vi "CAN wait.vi"(4 "error in (no error)":errorcluster, 5 "Timeout":i32=1000, 6 "Cob ID":u32, 7 "CANopen in":refnum<class "CANopen.lvclass">) -> (0 "error out":errorcluster, 1 "Timeout?":bool, 2 "Data":variant, 3 "CANopen out":refnum<class "CANopen.lvclass">)   [LabVIEW 2017, in "canopen.lvlib" / "CANopen.lvclass"]
doc: "Waits until a specific COB-ID is sent or a specific timeout is elapsed. This VI is <B>blocking</B>!"
uses:
  CANopen.lvclass
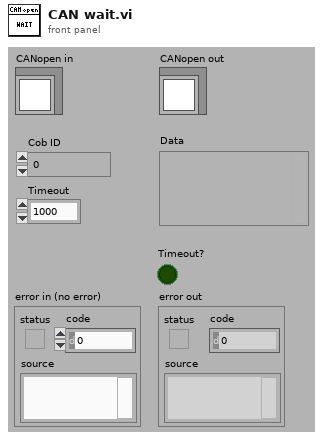
[diagram p1: front panel]
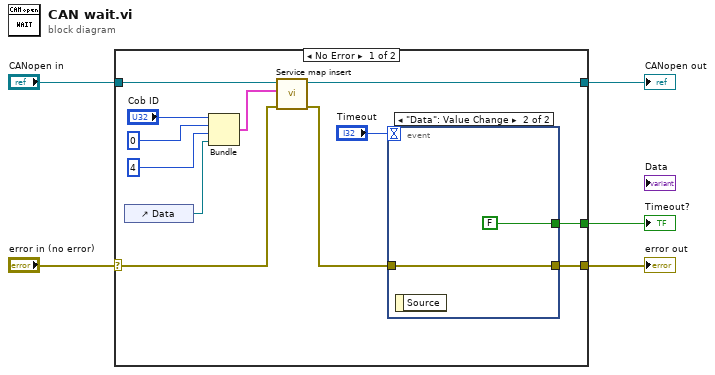
[diagram p0: block diagram]
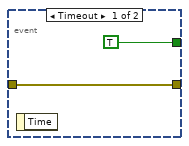
[diagram p2: hidden frame]
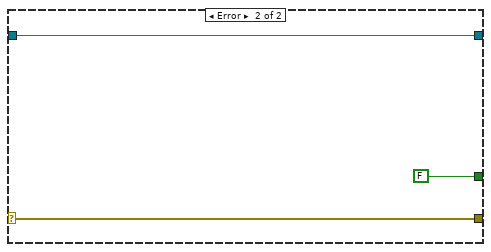
[diagram p3: hidden frame]
diagram:
  n1 = case shown="No Error" "error in (no error)" {
    selector: "error in (no error)" -> [w6 w23]
    tunnel: [w17 w24] -> w5
    tunnel: "CANopen in" -> [w11 w24]
    tunnel: [w8 w23] -> w3
    tunnel: [w7 FALSE ("Timeout?")] -> w2
    frame No Error {
      n2 = control-ref of="Data"() -> (w12:refnum<vi>)
      n3 = Bundle("Cob ID"="Cob ID", u8 0, u8 4, "Data"=w12) -> (w13:cluster{"Cob ID":u32, u8, u8, "Data":refnum<vi>})  [unwired: 1 out]
      n4 = call "Service map insert.vi"("error in (no error)"=w6, "Map entry"=w13, "CANopen in"=w11) -> ("error out"=w9:errorcluster, "CANopen out"=w17:refnum<class "CANopen.lvclass">)  [unwired: 3 out]
      n5 = event shown="[1] \"Data\": Value Change" {
        selector: _ -> [_ _]
        dyn-events: _ -> [_ _]
        timeout: "Timeout" -> [_ _]
        tunnel: w9 -> [w19 w21]
        tunnel: [w19 w21] -> w8
        tunnel: [TRUE ("Timeout?") FALSE ("Timeout?")] -> w7
        event Timeout {
          n6 = event-data() -> ()  [unwired: 2 out]
        }
        event "Data": Value Change {
          n7 = event-data() -> ()  [unwired: 2 out]
        }
      }
    }
    frame Error {
    }
  }
  "error out" <- w3
  "CANopen out" <- w5
  "Timeout?" <- w2
